vi "RT Driver VI.vi"(7 "Operation":T1, 11 "Device Reference in":T2 format="%.0x") -> (0 "Error Code":i32)   [LabVIEW 2019, in "MD4Logger Engine.lvlib"]
uses:
  MD4Logger Engine.lvlib
  <vilib>/NI VeriStand/Custom Device API/Custom Device Item Ref.ctl
  <vilib>/NI VeriStand/Custom Device API/Hardware Interface Driver VI Operation.ctl
  Shared/Compiled.Settings.ctl
  RTStateVariables.ctl
  <vilib>/NI/NIVS Inline Async API/_VS Inline Async API/VS Inline Async API/VS Inline Async API.lvclass
  <vilib>/NI VeriStand/Custom Device API/Custom Device Channel Type.ctl
  <vilib>/NI/NIVS Inline Async API/_VS Inline Async API/VS Inline Async API/VS Inline Async API.lvclass/VS Inline Async API.ctl
  <vilib>/NI/NIVS Inline Async API/_Data Access Engine/Data Access Engine/Data Access Engine.lvclass/Data Access Engine.ctl
  <vilib>/NI/NIVS Inline Async API/_Data Access Engine/Access Type Classes/Write/Write.lvclass/Write.ctl
  <vilib>/NI/NIVS Inline Async API/_Data Access Engine/Access Type Classes/ReadWrite/ReadWrite.lvclass/ReadWrite.ctl
  <vilib>/NI/NIVS Inline Async API/_Data Access Engine/Access Type Classes/Read/Read.lvclass/Read.ctl
  <vilib>/NI/NIVS Inline Async API/_Data Access Engine/Data Access Engine/Methods/Data.Engine.Read Data from HW.vi
  <vilib>/NI/NIVS Inline Async API/_VS Inline Async API/Error Handling Process/SubVIs/Error.GetError.vi
  <vilib>/NI/NIVS Inline Async API/_Data Access Engine/Data Access Engine/Methods/Data.Engine.Write Data to HW.vi
  <vilib>/NI/NIVS Inline Async API/_Data Access Engine/Access Type Classes/ReadWrite/ReadWrite.EngineData.vi
  <vilib>/NI/NIVS Inline Async API/_Data Access Engine/Access Type Classes/Write/Write.EngineData.vi
  <vilib>/NI/NIVS Inline Async API/_Data Access Engine/Access Type Classes/Read/Read.EngineData.vi
  <vilib>/NI VeriStand/Custom Device API/NI VeriStand - Get Channel Value by Data Reference.vi
  <vilib>/NI VeriStand/Custom Device API/NI VeriStand - Set Channel Value by Data Reference.vi
  <vilib>/NI VeriStand/Custom Device API/NI VeriStand - Get Channel Values by Block Data Reference.vi
  Shared/Constants.vi
  <vilib>/NI VeriStand/Custom Device Tools/Custom Device Utility Library/NI VeriStand - Search for Item by GUID.vi
  <vilib>/NI VeriStand/Custom Device API/Get Item Property (Path).vi
  <vilib>/NI VeriStand/Custom Device API/Global Data Refs.vi
  <vilib>/NI VeriStand/Custom Device API/Custom Device API.lvlib
  <vilib>/NI VeriStand/Custom Device Tools/Custom Device Utility Library/Custom Device Utility Library.lvlib
  Shared/MD4Logger Shared.lvlib
  <vilib>/NI VeriStand/Custom Device API/Set Item Property (Variant).vi
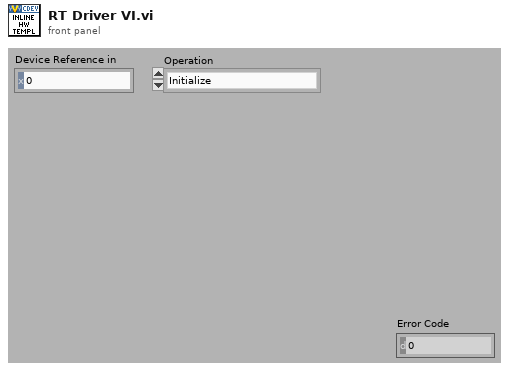
[diagram p1: front panel]
types:
  T1 = typedef "Custom Device API.lvlib/Hardware Interface Driver VI Operation.ctl" = enum16{"Initialize", "Start", "Read Data from HW", "Write Data to HW", "Close"}
  T2 = typedef "Custom Device API.lvlib/Custom Device Item Ref.ctl" = u64
  T3 = typedef "MD4Logger Engine.lvlib/RTStateVariables.ctl" = cluster{"Async":refnum<class "VS Inline Async API.lvclass">, "Settings":T4}
  T4 = typedef "MD4Logger Shared.lvlib/Compiled.Settings.ctl" = cluster{"Name":string, "Folder Path":path, "Channnel Names":cluster{"Name":string, "Unit":string}[]}
  T5 = typedef "Custom Device API.lvlib/Custom Device Channel Type.ctl" = enum16{"Input", "Output"}
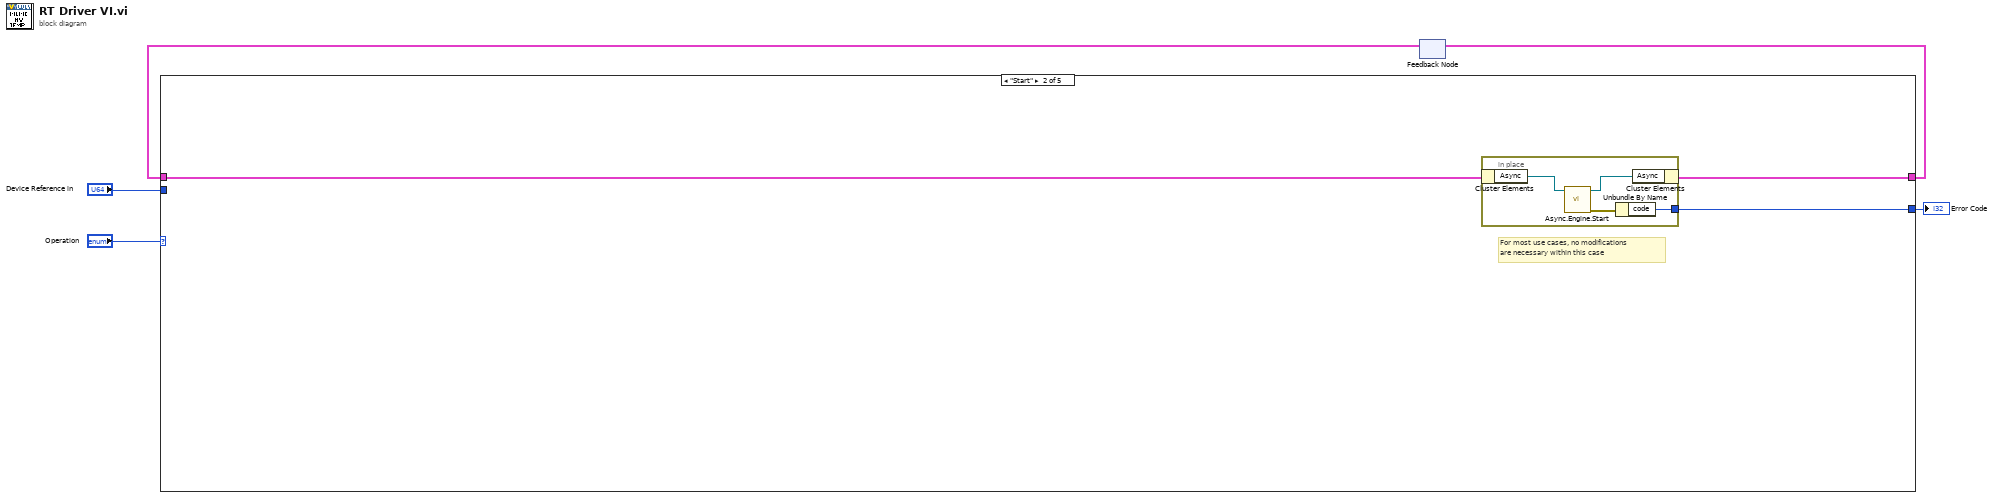
[diagram p0: block diagram]
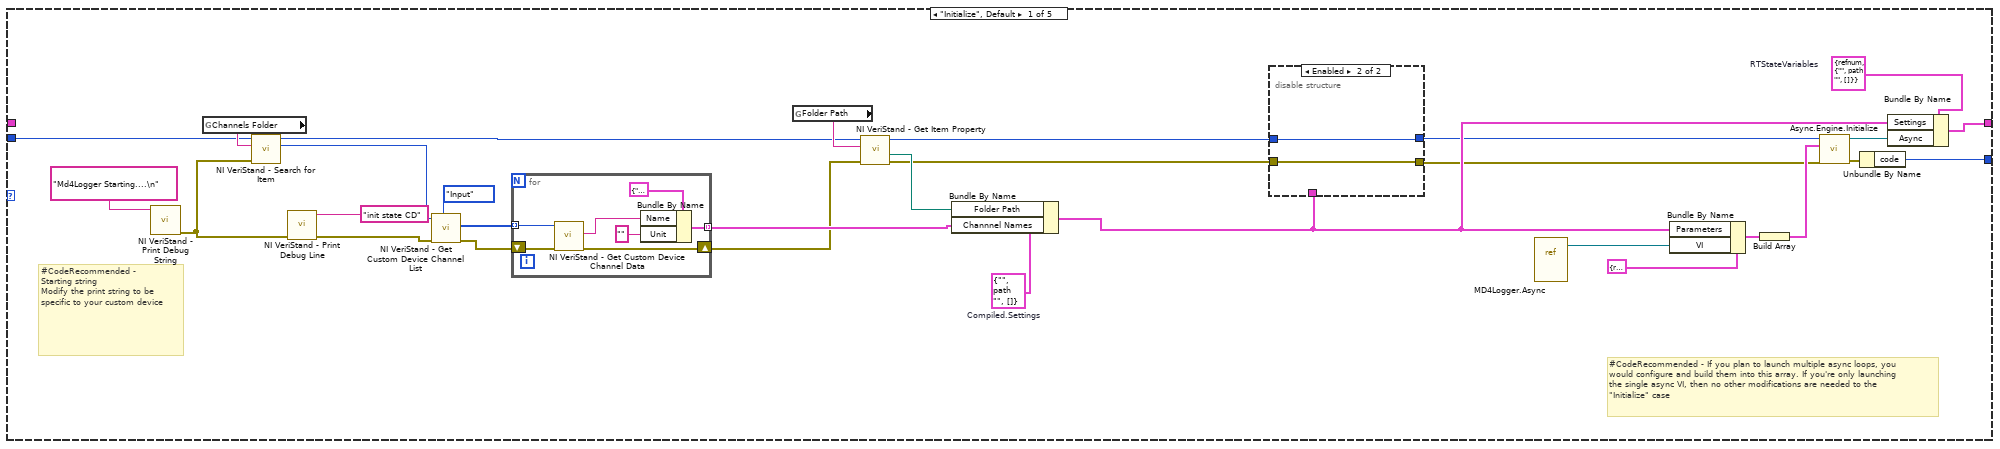
[diagram p2: hidden frame]
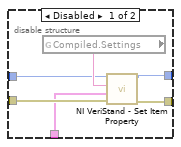
[diagram p3: hidden frame]
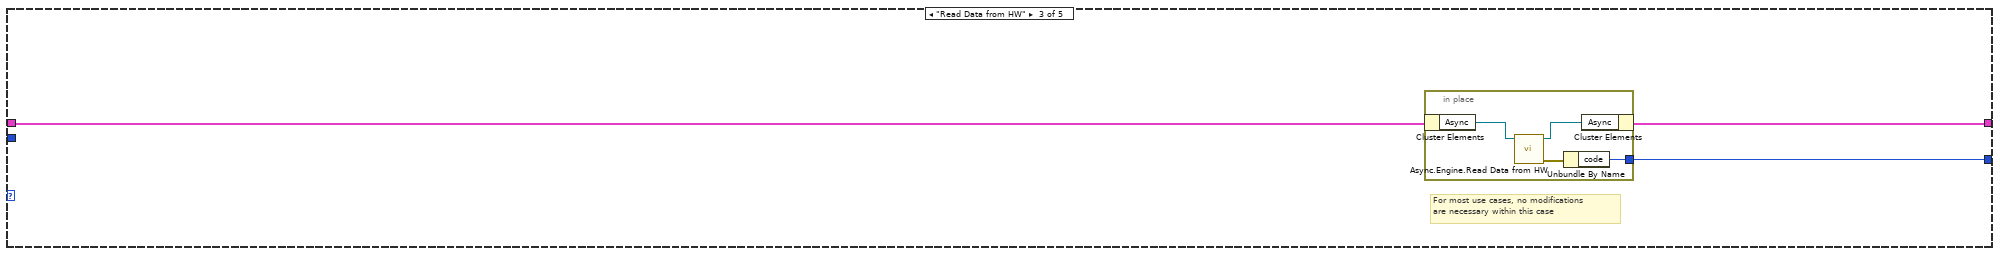
[diagram p4: hidden frame]
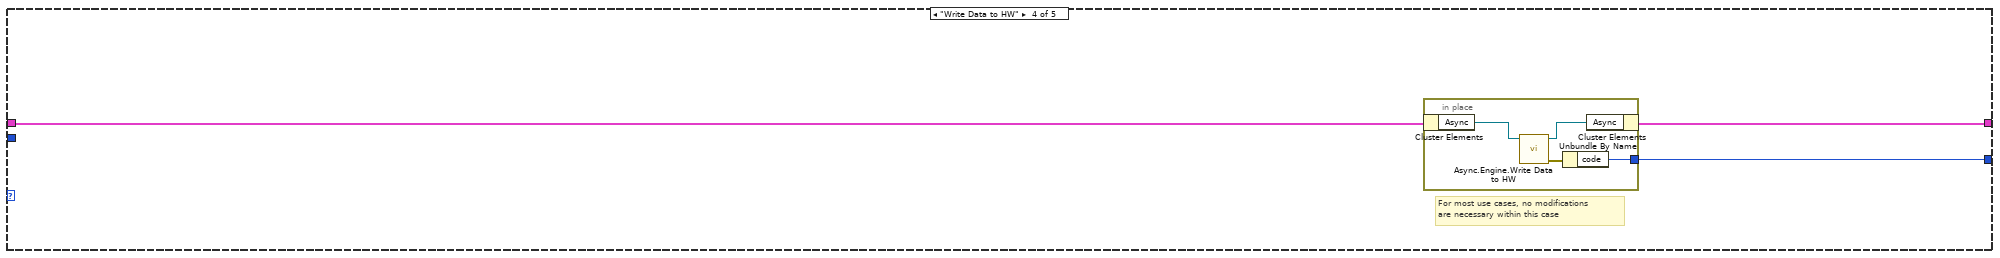
[diagram p5: hidden frame]
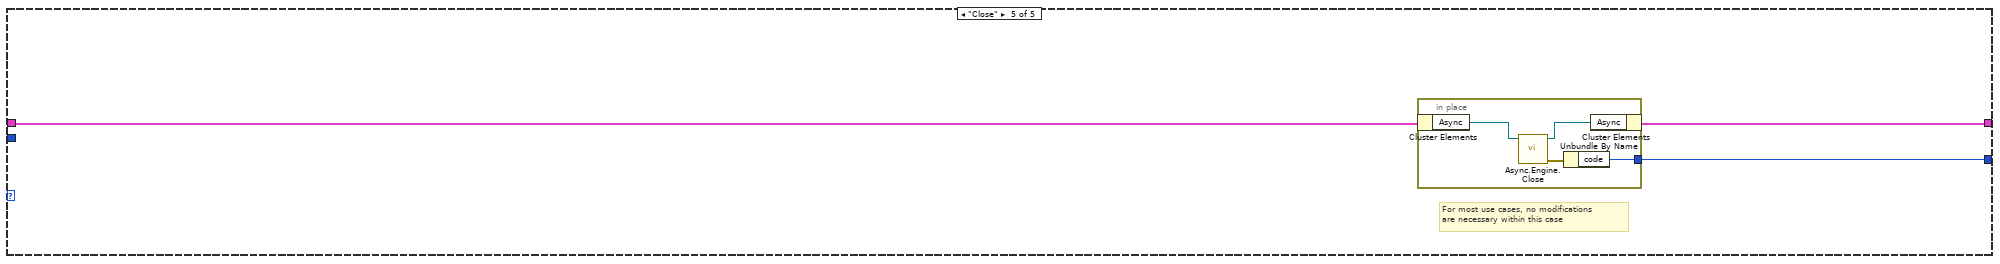
[diagram p6: hidden frame]
diagram:
  n1 = feedback #1() -> (w3:T3)  [unwired: 1 out]
  n2 = case shown="\"Start\"" "Operation" {
    tunnel: [w33 w53 w58 w65 w73] -> w4
    tunnel: w3 -> [_ w51 w60 w66 w74]
    tunnel: "Device Reference in" -> [w20 _ _ _ _]
    tunnel: [w35 w52 w59 w67 w72] -> w1
    frame "Initialize", Default {
      w29 = T3 {"Async"=refnum, "Settings"={"Name"="", "Folder Path"=path "", "Channnel Names"=[]}}  # RTStateVariables
      w24 = T4 {"Name"="", "Folder Path"=path "", "Channnel Names"=[]}  # Compiled.Settings
      # "#CodeRecommended - Starting string\nModify the print string to be specific to your custom device"
      # "#CodeRecommended - If you plan to launch multiple async loops, you would configure and build them into this array. If you're only launching the single async VI, then no other modifications are needed to the \"Initialize\" case"
      n3 = call <vilib>:"NI VeriStand - Print Debug String.vi"("Message"="Md4Logger Starting....\n") -> ("error out"=w7:errorcluster)  [unwired: 10 in]
      n4 = global read "Constants.vi" "Channels Folder"() -> (w21:string)
      n5 = call-poly <vilib>:"NI VeriStand - Search for Item.vi"("error in"=w7, "Item GUID"=w21, "Section Ref in"=w20) -> ("Item Ref"=w19:T2, "Section Ref out"=w16:T2)  [unwired: 5 in, 2 out]
      n6 = call <vilib>:"NI VeriStand - Print Debug Line.vi"("error in (no error)"=w7, "Message"="init state CD") -> ("error out"=w6:errorcluster)  [unwired: 9 in]
      n7 = call <vilib>:"NI VeriStand - Get Custom Device Channel List.vi"("Channel Type"=Custom_Device_Channel_Type."Input", "error in (no error)"=w6, "Device Ref in"=w19) -> ("error out"=w14:errorcluster, "Specified Channel Ref List"=w17:T2[])  [unwired: 6 in, 1 out]
      n8 = for {
        tunnel: w17 -> [w50] mode=indexing
        tunnel: [w46] -> w15 mode=indexing
        shift-right: [w44] -> w13
        shift-left: w14 -> [w45]
        n9 = call <vilib>:"NI VeriStand - Get Custom Device Channel Data.vi"("error in (no error)"=w45, "Channel Ref in"=w50) -> ("error out"=w44:errorcluster, "Channel Name"=w48:string)  [unwired: 4 in, 4 out]
        n10 = Bundle By Name(cluster=cluster{"Name":string, "Unit":string} {"Name"="", "Unit"=""} ("Channel"), "Name"=w48, "Unit"="") -> (w46:cluster{"Name":string, "Unit":string})
      }
      n11 = global read "Constants.vi" "Folder Path"() -> (w25:string)
      n12 = call-poly <vilib>:"NI VeriStand - Get Item Property.vi"("error in (no error)"=w13, "Property Name"=w25, "Item Ref in"=w16) -> ("error out"=w22:errorcluster, "Value"=w23:path, "Item Ref out"=w9:T2)  [unwired: 5 in, 1 out]
      n13 = Bundle By Name(cluster=w24, "Folder Path"=w23, "Channnel Names"=w15) -> (w12:T4)
      n14 = disable-structure shown="Enabled" {
        disable-tunnel: w22 -> [w41 w42]
        disable-tunnel: w12 -> [w39 _]
        disable-tunnel: [w38 w42] -> w11
        disable-tunnel: [w37 w43] -> w10
        disable-tunnel: w9 -> [w36 w43]
        frame Disabled {
          n15 = global read "Constants.vi" "Compiled.Settings"() -> (w40:string)
          n16 = call-poly <vilib>:"NI VeriStand - Set Item Property.vi"("error in (no error)"=w41, "Value"=w39, "Property Name"=w40, "Item Ref in"=w36) -> ("error out"=w38:errorcluster, "Item Ref out"=w37:T2)  [unwired: 5 in, 1 out]
        }
        frame Enabled {
        }
      }
      n17 = vi-ref "MD4Logger.Async.vi"() -> (w26:refnum<vi>)
      n18 = Bundle By Name(cluster=cluster{"VI":refnum<vi>, "Parameters":variant} {"VI"=refnum, "Parameters"=variant} ("Process"), "Parameters"=w12, "VI"=w26) -> (w31:cluster{"VI":refnum<vi>, "Parameters":variant})
      n19 = Build Array(w31) -> (w28:cluster{"VI":refnum<vi>, "Parameters":variant}[])
      n20 = call <vilib>:"Async.Engine.Initialize.vi"("error in (no error)"=w11, "Processes"=w28, "Custom Device Ref"=w10) -> ("error out"=w30:errorcluster, "Async"=w34:refnum<class "VS Inline Async API.lvclass">)  [unwired: 7 in]
      n21 = Unbundle By Name(w30) -> ("code"=w35:i32)
      n22 = Bundle By Name(cluster=w29, "Settings"=w12, "Async"=w34) -> (w33:T3)
    }
    frame "Start" {
      # "For most use cases, no modifications \nare necessary within this case"
      n23 = in-place {
        in-place-border: [w54] -> w52
        n24 = in-place-cluster #2(w51) -> ("Async"=w57:refnum<class "VS Inline Async API.lvclass">)
        n25 = call <vilib>:"Async.Engine.Start.vi"("VS Inline Async API in"=w57) -> ("error out"=w55:errorcluster, "VS Inline Async API out"=w56:refnum<class "VS Inline Async API.lvclass">)  [unwired: 9 in]
        n26 = Unbundle By Name(w55) -> ("code"=w54:i32)
        n27 = in-place-cluster #2("Async"=w56) -> (w53:T3)
      }
    }
    frame "Read Data from HW" {
      # "For most use cases, no modifications \nare necessary within this case"
      n28 = in-place {
        in-place-border: [w62] -> w59
        n29 = in-place-cluster #3(w60) -> ("Async"=w64:refnum<class "VS Inline Async API.lvclass">)
        n30 = call <vilib>:"Async.Engine.Read Data from HW.vi"("Async in"=w64) -> ("error out"=w61:errorcluster, "Async out"=w63:refnum<class "VS Inline Async API.lvclass">)  [unwired: 9 in]
        n31 = Unbundle By Name(w61) -> ("code"=w62:i32)
        n32 = in-place-cluster #3("Async"=w63) -> (w58:T3)
      }
    }
    frame "Write Data to HW" {
      # "For most use cases, no modifications \nare necessary within this case"
      n33 = in-place {
        in-place-border: [w71] -> w67
        n34 = in-place-cluster #4(w66) -> ("Async"=w69:refnum<class "VS Inline Async API.lvclass">)
        n35 = call <vilib>:"Async.Engine.Write Data to HW.vi"("VS Inline Async API in"=w69) -> ("error out"=w70:errorcluster, "VS Inline Async API out"=w68:refnum<class "VS Inline Async API.lvclass">)  [unwired: 9 in]
        n36 = Unbundle By Name(w70) -> ("code"=w71:i32)
        n37 = in-place-cluster #4("Async"=w68) -> (w65:T3)
      }
    }
    frame "Close" {
      # "For most use cases, no modifications \nare necessary within this case"
      n38 = in-place {
        in-place-border: [w76] -> w72
        n39 = in-place-cluster #5(w74) -> ("Async"=w78:refnum<class "VS Inline Async API.lvclass">)
        n40 = call <vilib>:"Async.Engine.Close.vi"("Async in"=w78) -> ("error out"=w75:errorcluster, "Async out"=w77:refnum<class "VS Inline Async API.lvclass">)  [unwired: 9 in]
        n41 = Unbundle By Name(w75) -> ("code"=w76:i32)
        n42 = in-place-cluster #5("Async"=w77) -> (w73:T3)
      }
    }
  }
  "Error Code" <- w1
  n43 = feedback-in #1(w4) -> ()
